vi "Tachomodus (SubVI).vi"(7 "cvt":bool, 8 "Leistung":refnum<vi>, 9 "Stopp":refnum<vi>, 10 "Hinterrad":refnum<vi>, 11 "Welle":refnum<vi>) -> ()   [LabVIEW 2014]
panel:
  in  "Text Rolle":string
  in  "Text Zündung":string
  out "Welle [1/min]\n[1/min]":cluster{u16, u16}(knob) caption="Welle\n[1/min]" scale=0.0..60000.0
  out "Hinterrad (Tacho)\n[km/h]":u16(knob) caption="Hinterrad\n[km/h]" scale=0.0..150.0 scale format="%#.0f"
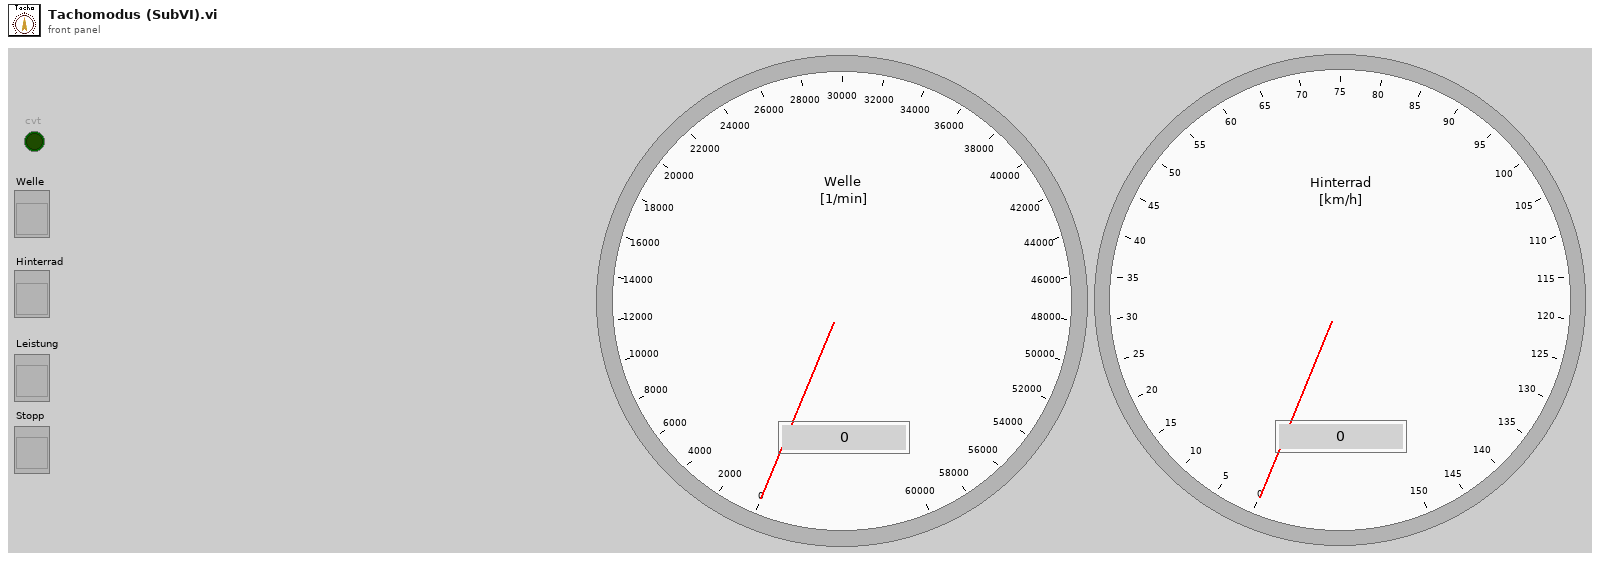
[diagram p1: front panel]
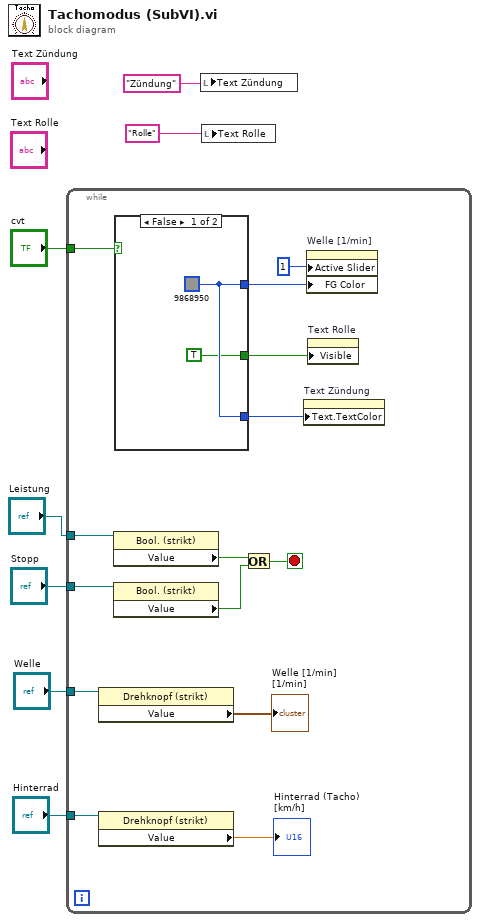
[diagram p0: block diagram]
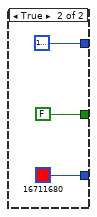
[diagram p2: hidden frame]
diagram:
  n1 = while {
    tunnel: "Welle" -> [w21]
    tunnel: "Hinterrad" -> [w20]
    tunnel: "Leistung" -> [w19]
    tunnel: "Stopp" -> [w17]
    tunnel: "cvt" -> [w12]
    stop <- w16 stop-if-true
    n2 = property class="Drehknopf (strikt)"(reference=w21) -> ("Value"=→"Welle [1/min]\n[1/min]":cluster{dbl, dbl})  [unwired: 1 in, 2 out]
    n3 = property class="Drehknopf (strikt)"(reference=w20) -> ("Value"=→"Hinterrad (Tacho)\n[km/h]":dbl)  [unwired: 1 in, 2 out]
    n4 = property class="Bool. (strikt)"(reference=w19) -> ("Value"=w18:bool)  [unwired: 1 in, 2 out]
    n5 = property class="Bool. (strikt)"(reference=w17) -> ("Value"=w15:bool)  [unwired: 1 in, 2 out]
    n6 = case shown="False" w12 {
      tunnel: [w23 u32 16711680] -> w11
      tunnel: [w23 u32 16777216] -> w9
      tunnel: [TRUE FALSE] -> w8
      frame False {
        w23 = u32 9868950
      }
      frame True {
      }
    }
    n7 = Or(x=w18, y=w15) -> (x .or. y?=w16:bool)
    n8 = property on="Text Zündung" class="Str"("Text.TextColor"=w11) -> ()  [unwired: 2 in, 2 out]
    n9 = property on="Welle [1/min]" class="Drehknopf (strikt)"("Active Slider"=1, "FG Color"=w9) -> ()  [unwired: 2 in, 2 out]
    n10 = property on="Text Rolle" class="Str"("Visible"=w8) -> ()  [unwired: 2 in, 2 out]
  }
  n11 = local write "Text Zündung"("Zündung") -> ()
  n12 = local write "Text Rolle"("Rolle") -> ()
